vi "PH_PILS.enable Laser.vi"(0 "i ref in":refnum<vi>, 5 "error in":errorcluster) -> (14 "i ref out":refnum<vi>, 19 "error out":errorcluster)   [LabVIEW 2014, in "PH_PILS.lvlib"]
uses:
  PH_PILS.lvlib
  PH_Common/PH_Common.lvlib
  PH_SystemInformation/PH_SystemInformation.lvlib
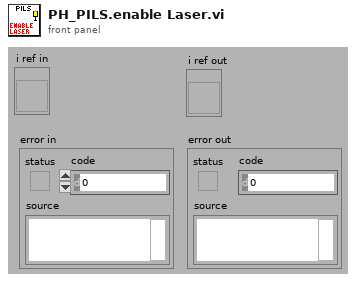
[diagram p1: front panel]
types:
  T1 = typedef "PH_PILS.lvlib/PH_PILS.i attribute.ctl" = cluster{"Boolean":cluster{"GUI Ref":refnum<vi>, "Status":i32}[], "GUI Refs Exp. Shutters":cluster{"1":refnum<vi>, "2":refnum<vi>, "3":refnum<vi>, "4":refnum<vi>}, "Tristate2Run GUI Refs":refnum<vi>[], "EO-Likes":cluster{"GUI Ref":refnum<vi>, "Status":i32}[], "Operation Mode":cluster{"Operation Mode":T2, "GUI":cluster{"Ref State":refnum<vi>, "Ref":refnum<vi>}, "Servicemode":cluster{"Tagname":string, "Status":i32}, "Labormode":cluster{"Tagname":string, "Status":i32}, "Searchmode":cluster{"Tagname":string, "Status":i32}, "Shotmode":cluster{"Tagname":string, "Status":i32}}, "Submode":cluster{"Submode":T3, "GUI":cluster{"Ref State":refnum<vi>, "Ref":refnum<vi>}, "Submode":cluster{"Tagname":string, "Status":i32}}, "Experiment":cluster{"Experiment":enum16{"unknown", "intern", "4 (Z6)", "3", "2", "1"}, "GUI":cluster{"Ref State":refnum<vi>, "Ref":refnum<vi>}, "intern":cluster{"Tagname":string, "Status":i32}, "Exp 4":cluster{"Tagname":string, "Status":i32}, "Exp 3":cluster{"Tagname":string, "Status":i32}, "Exp 2":cluster{"Tagname":string, "Status":i32}, "Exp 1":cluster{"Tagname":string, "Status":i32}}, "TristateNormal":cluster{"GUI Ref":refnum<vi>, "Status":i32}[], "Door Tags":cluster{"GUI Ref":refnum<vi>, "Status":i32}[], "GUIlessTags":cluster{"Name":string, "Status":i32}[], "Beamline GUI Refs":refnum<vi>[], "Special Boolean":cluster{"GUI Ref":refnum<vi>, "Status":i32}[], "Laserpower":cluster{"GUI Ref":refnum<vi>, "Status":i32}[], "Shutter":cluster{"GUI Ref":refnum<vi>, "Status":i32}[], "Tristate EO Like":cluster{"GUI Ref":refnum<vi>, "Status":i32}[], "PP":cluster{"GUI Ref":refnum<vi>, "Status":i32, "Head Ref":refnum<vi>, "Slider Ref":refnum<vi>}[], "Switch Knobs":cluster{"GUI Ref":refnum<vi>, "Status":i32}[], "Latch Knob GUI Refs":refnum<vi>[], "FailureCounter":i32, "Enabled Status":cluster{"Laser":i32, "PreAmp":i32, "MainAmp":i32}, "Mercury":refnum<vi>, "Instance Rods":string, "Logfile":path, "Beckhoff-Instance Internal":string, "Beckhoff-Instance External":string, "Enabling Rights":cluster{"Name":string, "Password":string, "PA?":bool, "MA?":bool, "Exp?":bool}[]}
  T2 = typedef "PH_PILS.lvlib/PH_PILS.Operation Mode.ctl" = enum16{"unknown", "Service", "Labor", "Search", "Shot"}
  T3 = typedef "PH_PILS.lvlib/PH_PILS.Submode.ctl" = enum16{"unknown", "HV-Normal", "HV-Test"}
  T4 = enum16{"Laser", "PreAmp", "MainAmp", "Exp 1", "Exp 2", "Exp 3", "Exp 4"}
  T5 = typedef "PH_SystemInformation.lvlib/PH_SystemInformationEnabling State.ctl" = i32
  T6 = typedef "PH_SystemInformation.lvlib/PH_SystemInformation.i attribute.ctl" = cluster{"Laser Enabling":cluster{"GUI Ref":refnum<vi>, "Enabling State":T5}, "PreAmp Enabling":cluster{"GUI Ref":refnum<vi>, "Enabling State":T5}, "MainAmp Enabling":cluster{"GUI Ref":refnum<vi>, "Enabling State":T5}, "Emergency Off":cluster{"GUI Ref":refnum<vi>, "State":enum16{"no info", "off/false", "Alarm"}}, "Enabling Exp. 1":cluster{"GUI Ref":refnum<vi>, "Enabling State":T5}, "Enabling Exp. 2":cluster{"GUI Ref":refnum<vi>, "Enabling State":T5}, "Enabling Exp. 3":cluster{"GUI Ref":refnum<vi>, "Enabling State":T5}, "Enabling Exp. 4":cluster{"GUI Ref":refnum<vi>, "Enabling State":T5}, "Timing Mode":cluster{"GUI Ref":refnum<vi>, "PHELIX_Timing_Mode":enum32{"10 Hz", "0.5 Hz", "Shot"}}}
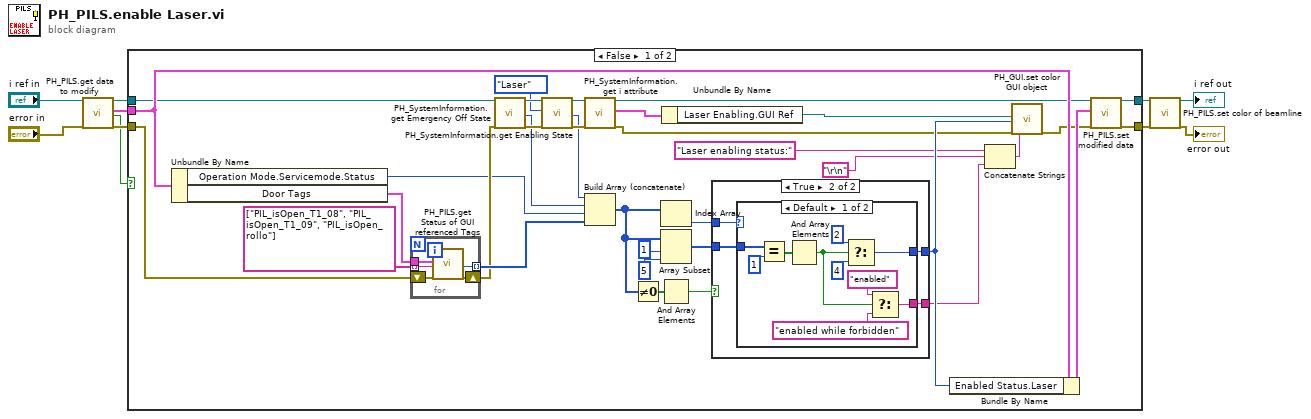
[diagram p0: block diagram]
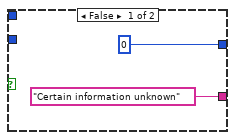
[diagram p2: hidden frame]
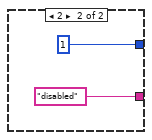
[diagram p3: hidden frame]
diagram:
  n1 = call "PH_PILS.get data to modify.vi"("i ref in"="i ref in", "error in (no error)"="error in") -> ("i ref out"=w6:refnum<vi>, "i attribute"=w7:T1, "timed out"=w5:bool, "error out"=w9:errorcluster)  [unwired: 14 in]
  n2 = case shown="False" w5 {
    tunnel: w9 -> [w39 w69]
    tunnel: w7 -> [w38 _]
    tunnel: [w42 w69] -> w3
    tunnel: w6 -> [w31 w70]
    tunnel: [w41 w70] -> w4
    frame False {
      n3 = Unbundle By Name(w38) -> ("Operation Mode.Servicemode.Status"=w15:i32, "Door Tags"=w19:cluster{"GUI Ref":refnum<vi>, "Status":i32}[])
      n4 = for {
        tunnel: string[] ["PIL_isOpen_T1_08", "PIL_isOpen_T1_09", "PIL_isOpen_rollo"] -> [w67] mode=indexing
        tunnel: [w68] -> w45 mode=indexing
        shift-right: [w66] -> w17
        shift-left: w39 -> [w65]
        tunnel: w19 -> [w64]
        n5 = call "PH_PILS.get Status of GUI referenced Tags.vi"("Tags"=w64, "Tagname"=w67, "error in"=w65) -> ("Status"=w68:i32, "error out"=w66:errorcluster)  [unwired: 13 in, 2 out]
      }
      n6 = call "PH_SystemInformation.get Emergency Off State.vi"("i ref in"=w31, "error in (no error)"=w17) -> ("i ref out"=w23:refnum<vi>, "Emergency Off State"=w20:enum16{"no info", "off/false", "Alarm"}, "error out"=w22:errorcluster)  [unwired: 15 in]
      n7 = call "PH_SystemInformation.get Enabling State.vi"("i ref in"=w23, "Wanted State"=T4."Laser", "error in (no error)"=w22) -> ("i ref out"=w29:refnum<vi>, "Enabling State"=w16:T5, "error out"=w25:errorcluster)  [unwired: 14 in]
      n8 = call "PH_SystemInformation.get i attribute.vi"("i ref in"=w29, "error in (no error)"=w25) -> ("i ref out"=w28:refnum<vi>, "i attribute"=w27:T6, "error out"=w24:errorcluster)  [unwired: 15 in]
      n9 = Build Array (concatenate)(w16, w20, w15, w45) -> (w32:T5[])
      n10 = Not Equal To 0?(x=w32) -> (x != 0?=w44:bool[])
      n11 = Index Array(array=w32) -> (element=w36:T5)  [unwired: 1 in]
      n12 = Array Subset(array=w32, index=1, length=5) -> (w33:T5[])
      n13 = And Array Elements(Boolean array=w44) -> (logical AND=w43:bool)
      n14 = Unbundle By Name(w27) -> ("Laser Enabling.GUI Ref"=w26:refnum<vi>)
      n15 = case shown="True" w43 {
        tunnel: [0 ("Status") w51] -> w37
        tunnel: w36 -> [_ w50]
        tunnel: w33 -> [_ w49]
        tunnel: ["Certain information unknown" w48] -> w11
        frame False {
        }
        frame True {
          n16 = case shown="Default" w50 {
            tunnel: [w56 1 ("y")] -> w51
            tunnel: w49 -> [w61 _]
            tunnel: [w53 "disabled"] -> w48
            frame Default {
              n17 = Equal?(x=w61, y=1) -> (x = y?=w59:bool[])
              n18 = And Array Elements(Boolean array=w59) -> (logical AND=w52:bool)
              n19 = Select(t=2 ("y"), s=w52, f=4 ("y")) -> (s? t:f=w56:i32)
              n20 = Select(t="enabled", s=w52, f="enabled while forbidden") -> (s? t:f=w53:string)
            }
            frame 2 {
            }
          }
        }
      }
      n21 = Bundle By Name(cluster=w38, "Enabled Status.Laser"=w37) -> (w40:T1)
      n22 = Concatenate Strings("Laser enabling status:", "\r\n", w11) -> (w12:string)
      n23 = call "PH_GUI.set color GUI object.vi"("GUI object Ref"=w26, "State"=w37, "error in (no error)"=w24, "Tip Strip (N/A)"=w12) -> ("error out"=w30:errorcluster)  [unwired: 15 in]
      n24 = call "PH_PILS.set modified data.vi"("i ref in"=w28, "i attribute"=w40, "error in (no error)"=w30) -> ("i ref out"=w41:refnum<vi>, "error out"=w42:errorcluster)  [unwired: 15 in]
    }
    frame True {
    }
  }
  n25 = call "PH_PILS.set color of beamline.vi"("i ref in"=w4, "error in"=w3) -> ("i ref out"=→"i ref out":refnum<vi>, "error out"=→"error out":errorcluster)  [unwired: 16 in]
